vi "Initialize Local Log.vi"(7 "LogLevel":T2, 8 "error in (no error)":errorcluster, 11 "Text File Configuration":T1={"Folder"=path "C:/", "Name"="Event Log", "Extension"="txt", "Max Size (MB)"=1, "Timestamp Filename"=TRUE}) -> (0 "error out":errorcluster, 3 "Logger out":refnum<class "Logger.lvclass">)   [LabVIEW 2020, in "Event Log.lvlib" / "Logger.lvclass"]
uses:
  Logger.lvclass
  <vilib>/gpm_packages/@cs/event-logger/Source/Composed Log/Types/Log Level.ctl
  <vilib>/gpm_packages/@cs/event-logger/Source/Text File Sink/Configuration.ctl
  <vilib>/gpm_packages/@cs/event-logger/Source/Composed Log/LoggerReference/LoggerReference.lvclass
  <vilib>/gpm_packages/@cs/event-logger/Source/Composed Log/LoggerReference/LoggerReference.lvclass/LoggerReference.ctl
  Logger.lvclass/Logger.ctl
  a570ed94-fdd8-4377-882c-dcf657bf05af.vi
  <vilib>/gpm_packages/@cs/event-logger/Source/Composed Log/LoggerReference/Return Aggregate Queues.vi
  <vilib>/gpm_packages/@cs/event-logger/Source/Composed Log/LoggerReference/Add Aggregate Log.vi
  a570ed94-fdd8-4377-882c-dcf657bf05af.vi/467b9aba-ab44-4297-978f-72bf0771973b.vi
  <vilib>/gpm_packages/@cs/event-logger/Source/Composed Log/LoggerReference/Send Add Sink.vi
  <vilib>/gpm_packages/@cs/event-logger/Source/Text File Sink/Text File Sink.lvclass
  C:/Program Files/National Instruments/LabVIEW 2020/vi.lib/gpm_packages/@cs/event-logger/Source/Composed Log/Log Sink/Log Sink.lvclass
  <vilib>/gpm_packages/@cs/event-logger/Source/Composed Log/Application Logger/Launch Worker Loop.vi
  <vilib>/gpm_packages/@cs/event-logger/Source/Composed Log/LoggerReference/Initialize Logger Instance.vi
  <vilib>/gpm_packages/@cs/event-logger/Source/Composed Log/IErrorFormat/IErrorFormat.lvclass
  <vilib>/gpm_packages/@cs/event-logger/Source/Composed Log/Log Sink/Log Sink.lvclass
  <vilib>/gpm_packages/@cs/event-logger/Source/Composed Log/Composed Log.lvlib
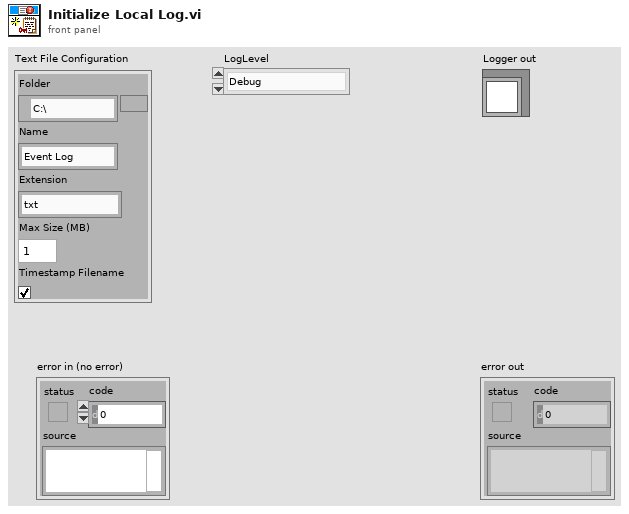
[diagram p1: front panel]
types:
  T1 = typedef "Text File Sink.lvclass/Configuration.ctl" = cluster{"Folder":path, "Name":string, "Extension":string, "Max Size (MB)":i64, "Timestamp Filename":bool}
  T2 = typedef "Composed Log.lvlib/Log Level.ctl" = enum16{"Debug", "Info", "Warning", "Error", "Critical"}
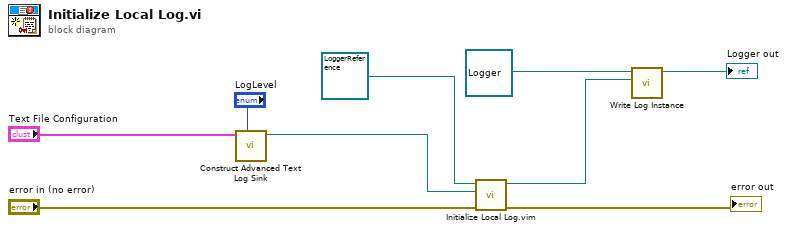
[diagram p0: block diagram]
diagram:
  n1 = call <vilib>:"Construct Advanced Text Log Sink.vi"("LogLevel"="LogLevel", "Text File Configuration"="Text File Configuration") -> ("Text File Sink out"=w6:refnum<class "Text File Sink.lvclass">)  [unwired: 9 in]
  n2 = call "Initialize Local Log.vim"("error in (no error)"="error in (no error)", "Startup Sink(s)"=w6, "Parent Log Reference"=refnum<class "LoggerReference.lvclass"> refnum) -> ("error out"=→"error out":errorcluster, "Log Instance Reference"=w5:refnum<class "LoggerReference.lvclass">)  [unwired: 6 in, 1 out]
  n3 = call "Write Log Instance.vi"("oggerReference."=w5, "Logger in"=refnum<class "Logger.lvclass"> refnum) -> ("Logger out"=→"Logger out":refnum<class "Logger.lvclass">)  [unwired: 9 in]
